vi "Module Identities.vi"(8 "error in (no error)":errorcluster, 11 "Historian Charting Manager in":refnum<class "Historian Charting Manager.lvclass">) -> (0 "error out":errorcluster, 2 "Identities":refnum<class "Identity.lvclass">[](array[class]), 3 "Historian Charting Manager out":refnum<class "Historian Charting Manager.lvclass">)   [LabVIEW 2020, in "VolatusGUI.lvlib" / "Historian Charting Manager.lvclass"]
uses:
  Historian Charting Manager.lvclass
  Volatus/Identity/Identity.lvclass
  Historian Charting Manager ID/Historian Charting Manager ID.lvclass
  C:/dev/lv20CE/relink/lv-volatus/Volatus/Identity/Identity.lvclass
  Historian Charting Manager.lvclass/Historian Charting Manager.ctl
  C:/dev/lv20CE/relink/lv-volatus/VolatusHistorian/Historian Charting Manager ID/Historian Charting Manager ID.lvclass
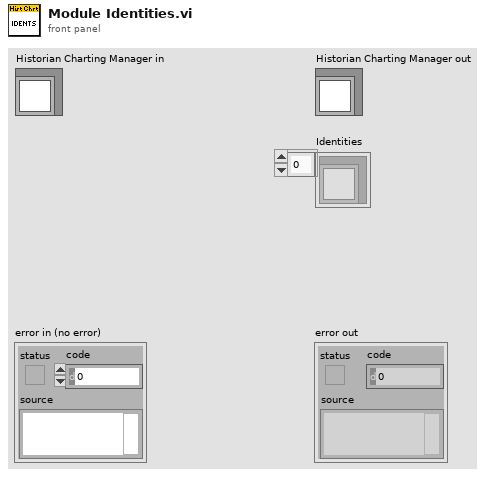
[diagram p1: front panel]
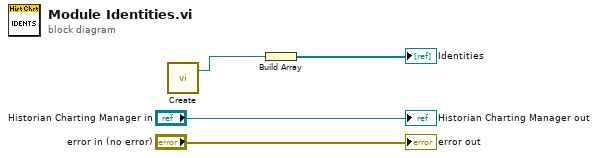
[diagram p0: block diagram]
diagram:
  n1 = call "Create.vi"() -> ("Historian Charting Manager ID out"=w2:refnum<class "Historian Charting Manager ID.lvclass">)  [unwired: 7 in]
  n2 = Build Array(w2) -> (→"Identities":refnum<class "Historian Charting Manager ID.lvclass">[])
  "error out" <- "error in (no error)"
  "Historian Charting Manager out" <- "Historian Charting Manager in"
